vi "TUNA forebrain SENSE.vi"(2 "error in":errorcluster, 4 "Boat Status":T1={"GPS"={"X pos"=0, "Y pos"=0, "Heading"=0.0}, "IR Sensors"=[{"Name"="Bow", "Angle"=0.0, "Distance"=0.0}], "MOT BAT"=7.2, "RIO BAT"=7.2}) -> (0 "error out":errorcluster, 1 "GPS":cluster{"X pos":i32, "Y pos":i32, "Heading":dbl})   [LabVIEW 2014]
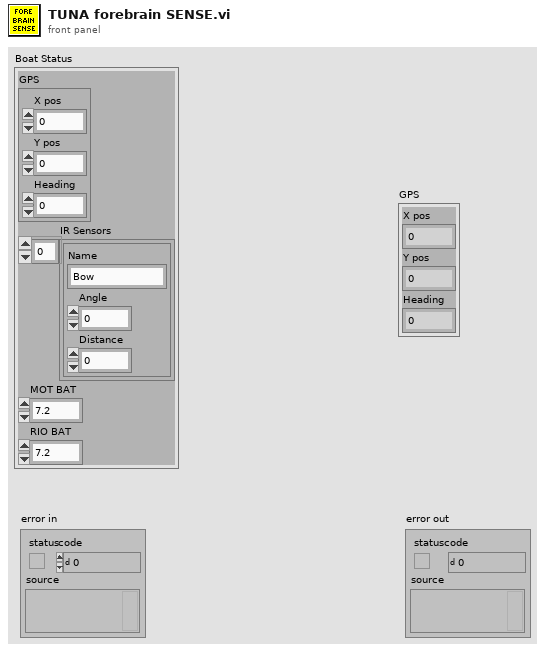
[diagram p1: front panel]
types:
  T1 = cluster{"GPS":cluster{"X pos":i32, "Y pos":i32, "Heading":dbl}, "IR Sensors":cluster{"Name":string, "Angle":dbl, "Distance":dbl}[], "MOT BAT":dbl, "RIO BAT":dbl}
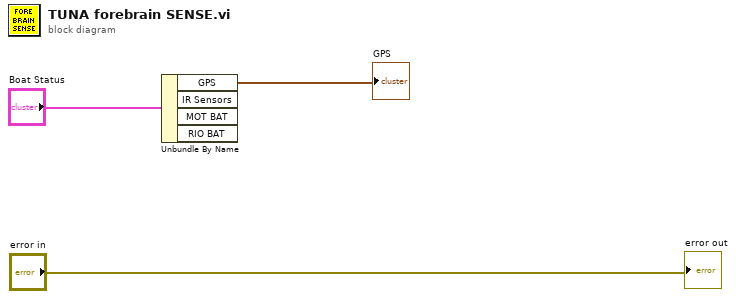
[diagram p0: block diagram]
diagram:
  n1 = Unbundle By Name("Boat Status") -> ("GPS"=→"GPS":cluster{"X pos":i32, "Y pos":i32, "Heading":dbl})  [unwired: 3 out]
  "error out" <- "error in"
